vi "Process Image.vi"(8 "error in (no error)":errorcluster, 10 "Image Analysis IN":T1, 11 "Cluster in":T3={"Crosshair IN"={"Draw"=TRUE, "Target"={"x"=20.0, "y"=20.0}, "Size"={"x"=20.0, "y"=20.0}, "Angle"=1250067.0, "Color"=1250067, "Thickness"=20, "CrosshairLabel"=""}, "Autoscale"=FALSE, "Scale"={"scale factor"=0.0, "Scale"=FALSE}, "Lowpass IN"={"LowPass"=FALSE, "Size & Tolerance"={"X Size"=0, "Y Size"=0, "% Tolerance"=0}}, "Image"=refnum, "GUI_centroid overlay"={"CentroidX array"=[], "CentroidY array"=[], "CentroidX"=0.0, "CentroidY"=0.0, "# images to average"=1250067, "Crosshair"={"Draw"=TRUE, "Target"={"x"=20.0, "y"=20.0}, "Size"={"x"=20.0, "y"=20.0}, "Angle"=1250067.0, "Color"=1250067, "Thickness"=20, "CrosshairLabel"=""}}, "GUI Crosshair"={"Draw"=TRUE, "Target"={"x"=20.0, "y"=20.0}, "Size"={"x"=20.0, "y"=20.0}, "Angle"=1250067.0, "Color"=1250067, "Thickness"=20, "CrosshairLabel"=""}, "Crosshair2 IN"={"Draw"=TRUE, "Target"={"x"=20.0, "y"=20.0}, "Size"={"x"=20.0, "y"=20.0}, "Angle"=1250067.0, "Color"=1250067, "Thickness"=20, "CrosshairLabel"=""}} {"Crosshair2 IN"."Thickness" max=0; "Crosshair2 IN"."Target"."y" min=0.0 max=0.0; "Crosshair2 IN"."Target"."x" min=0.0 max=0.0; "Crosshair2 IN"."Angle" format="%#_13g"; "Crosshair2 IN"."Size"."y" min=0.0 max=0.0; "Crosshair2 IN"."Size"."x" min=0.0 max=0.0; "GUI Crosshair"."Thickness" max=0; "GUI Crosshair"."Target"."y" min=0.0 max=0.0; "GUI Crosshair"."Target"."x" min=0.0 max=0.0; "GUI Crosshair"."Angle" format="%#_13g"; "GUI Crosshair"."Size"."y" min=0.0 max=0.0; "GUI Crosshair"."Size"."x" min=0.0 max=0.0; "GUI_centroid overlay"."Crosshair"."Thickness" max=0; "GUI_centroid overlay"."Crosshair"."Target"."y" min=0.0 max=0.0; "GUI_centroid overlay"."Crosshair"."Target"."x" min=0.0 max=0.0; "GUI_centroid overlay"."Crosshair"."Angle" format="%#_13g"; "GUI_centroid overlay"."Crosshair"."Size"."y" min=0.0 max=0.0; "GUI_centroid overlay"."Crosshair"."Size"."x" min=0.0 max=0.0; "Crosshair IN"."Thickness" max=0; "Crosshair IN"."Target"."y" min=0.0 max=0.0; "Crosshair IN"."Target"."x" min=0.0 max=0.0; "Crosshair IN"."Angle" format="%#_13g"; "Crosshair IN"."Size"."y" min=0.0 max=0.0; "Crosshair IN"."Size"."x" min=0.0 max=0.0}) -> (0 "error out":errorcluster, 2 "Image Analysis OUT":T1, 3 "Cluster out":T3={"Crosshair IN"={"Draw"=TRUE, "Target"={"x"=20.0, "y"=20.0}, "Size"={"x"=20.0, "y"=20.0}, "Angle"=1250067.0, "Color"=1250067, "Thickness"=20, "CrosshairLabel"=""}, "Autoscale"=FALSE, "Scale"={"scale factor"=0.0, "Scale"=FALSE}, "Lowpass IN"={"LowPass"=FALSE, "Size & Tolerance"={"X Size"=0, "Y Size"=0, "% Tolerance"=0}}, "Image"=refnum, "GUI_centroid overlay"={"CentroidX array"=[], "CentroidY array"=[], "CentroidX"=0.0, "CentroidY"=0.0, "# images to average"=1250067, "Crosshair"={"Draw"=TRUE, "Target"={"x"=20.0, "y"=20.0}, "Size"={"x"=20.0, "y"=20.0}, "Angle"=1250067.0, "Color"=1250067, "Thickness"=20, "CrosshairLabel"=""}}, "GUI Crosshair"={"Draw"=TRUE, "Target"={"x"=20.0, "y"=20.0}, "Size"={"x"=20.0, "y"=20.0}, "Angle"=1250067.0, "Color"=1250067, "Thickness"=20, "CrosshairLabel"=""}, "Crosshair2 IN"={"Draw"=TRUE, "Target"={"x"=20.0, "y"=20.0}, "Size"={"x"=20.0, "y"=20.0}, "Angle"=1250067.0, "Color"=1250067, "Thickness"=20, "CrosshairLabel"=""}} {"Crosshair2 IN"."Thickness" max=0; "Crosshair2 IN"."Target"."y" min=0.0 max=0.0; "Crosshair2 IN"."Target"."x" min=0.0 max=0.0; "Crosshair2 IN"."Angle" format="%#_13g"; "Crosshair2 IN"."Size"."y" min=0.0 max=0.0; "Crosshair2 IN"."Size"."x" min=0.0 max=0.0; "GUI Crosshair"."Thickness" max=0; "GUI Crosshair"."Target"."y" min=0.0 max=0.0; "GUI Crosshair"."Target"."x" min=0.0 max=0.0; "GUI Crosshair"."Angle" format="%#_13g"; "GUI Crosshair"."Size"."y" min=0.0 max=0.0; "GUI Crosshair"."Size"."x" min=0.0 max=0.0; "GUI_centroid overlay"."Crosshair"."Thickness" max=0; "GUI_centroid overlay"."Crosshair"."Target"."y" min=0.0 max=0.0; "GUI_centroid overlay"."Crosshair"."Target"."x" min=0.0 max=0.0; "GUI_centroid overlay"."Crosshair"."Angle" format="%#_13g"; "GUI_centroid overlay"."Crosshair"."Size"."y" min=0.0 max=0.0; "GUI_centroid overlay"."Crosshair"."Size"."x" min=0.0 max=0.0; "Crosshair IN"."Thickness" max=0; "Crosshair IN"."Target"."y" min=0.0 max=0.0; "Crosshair IN"."Target"."x" min=0.0 max=0.0; "Crosshair IN"."Angle" format="%#_13g"; "Crosshair IN"."Size"."y" min=0.0 max=0.0; "Crosshair IN"."Size"."x" min=0.0 max=0.0})   [LabVIEW 2013]
uses:
  Controls/Image Processing Controls.ctl
  Controls/Crosshair type def.ctl
  <vilib>/vision/Image Controls.llb/IMAQ Image.ctl
  Controls/GUI_running average centroid overlay.ctl
  Controls/Image Analysis Controls.ctl
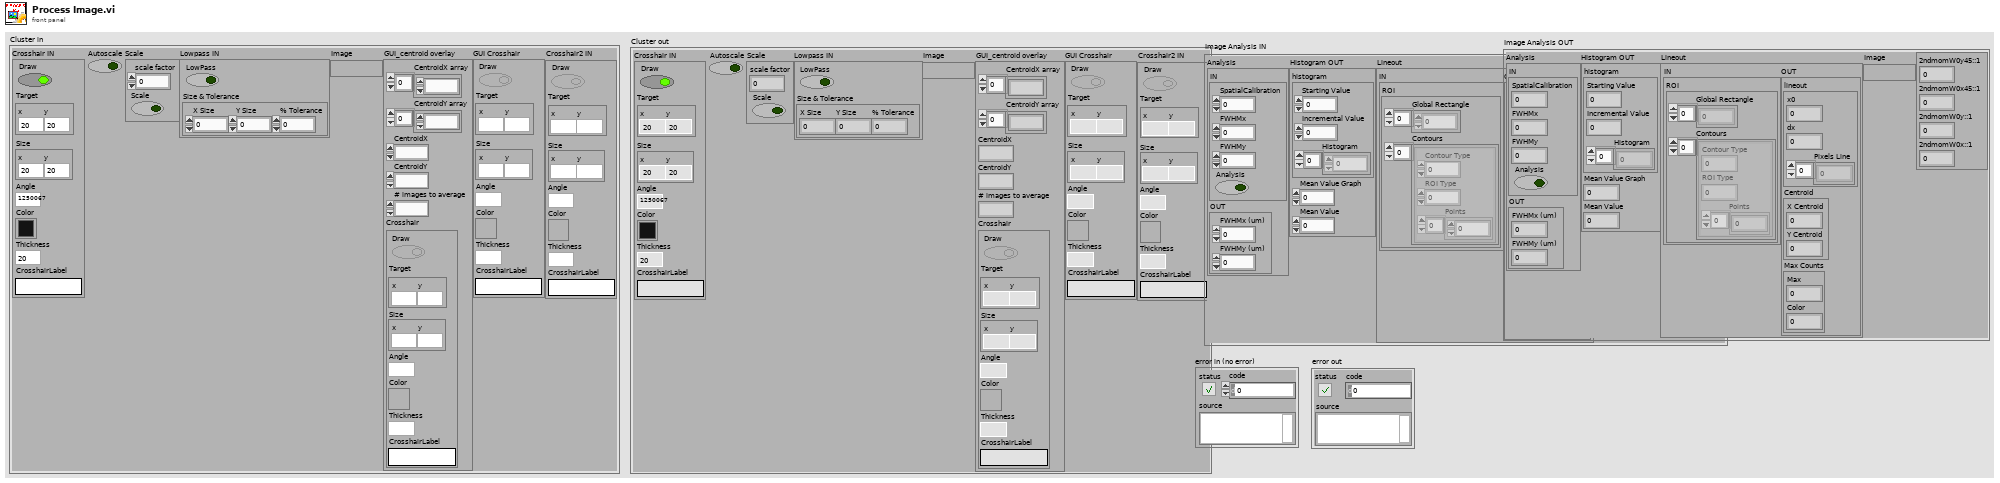
[diagram p1: front panel]
types:
  T1 = typedef "Image Analysis Controls.ctl" = cluster{"Analysis":cluster{"IN":cluster{"SpatialCalibration":dbl, "FWHMx":dbl, "FWHMy":dbl, "Analysis":bool}, "OUT":cluster{"FWHMx (um)":dbl, "FWHMy (um)":dbl}}, "Histogram OUT":cluster{"histogram":cluster{"Starting Value":sgl, "Incremental Value":sgl, "Histogram":u32[]}, "Mean Value Graph":sgl, "Mean Value":sgl}, "Lineout":cluster{"IN":cluster{"ROI":cluster{"Global Rectangle":i32[], "Contours":cluster{"Contour Type":u32, "ROI Type":u32, "Points":i32[]}[]}}, "OUT":cluster{"lineout":cluster{"x0":sgl, "dx":sgl, "Pixels Line":sgl[]}, "Centroid":cluster{"X Centroid":sgl, "Y Centroid":sgl}, "Max Counts":cluster{"Max":sgl, "Color":u32}}}, "Image":T2, "variables":cluster{"2ndmomW0y45::1":dbl, "2ndmomW0x45::1":dbl, "2ndmomW0y::1":dbl, "2ndmomW0x::1":dbl}}
  T2 = typedef "IMAQ Image.ctl" = refnum<image>
  T3 = typedef "Image Processing Controls.ctl" = cluster{"Crosshair IN":T4, "Autoscale":bool, "Scale":cluster{"scale factor":dbl, "Scale":bool}, "Lowpass IN":cluster{"LowPass":bool, "Size & Tolerance":cluster{"X Size":i32, "Y Size":i32, "% Tolerance":i32}}, "Image":T2, "GUI_centroid overlay":T5, "GUI Crosshair":T4, "Crosshair2 IN":T4}
  T4 = typedef "Crosshair type def.ctl" = cluster{"Draw":bool, "Target":cluster{"x":dbl, "y":dbl}, "Size":cluster{"x":dbl, "y":dbl}, "Angle":dbl, "Color":u32, "Thickness":u8, "CrosshairLabel":string}
  T5 = typedef "GUI_running average centroid overlay.ctl" = cluster{"CentroidX array":dbl[], "CentroidY array":dbl[], "CentroidX":dbl, "CentroidY":dbl, "# images to average":i32, "Crosshair":T4}
  T6 = cluster{"LowPass":bool, "Size & Tolerance":cluster{"X Size":i32, "Y Size":i32, "% Tolerance":i32}}
  T7 = cluster{"SpatialCalibration":dbl, "FWHMx":dbl, "FWHMy":dbl, "Analysis":bool}
  T8 = cluster{"ROI":cluster{"Global Rectangle":i32[], "Contours":cluster{"Contour Type":u32, "ROI Type":u32, "Points":i32[]}[]}}
  T9 = cluster{"histogram":cluster{"Starting Value":sgl, "Incremental Value":sgl, "Histogram":u32[]}, "Mean Value Graph":sgl, "Mean Value":sgl}
  T10 = cluster{"lineout":cluster{"x0":sgl, "dx":sgl, "Pixels Line":sgl[]}, "Centroid":cluster{"X Centroid":sgl, "Y Centroid":sgl}, "Max Counts":cluster{"Max Value":sgl, "Color":u32}}
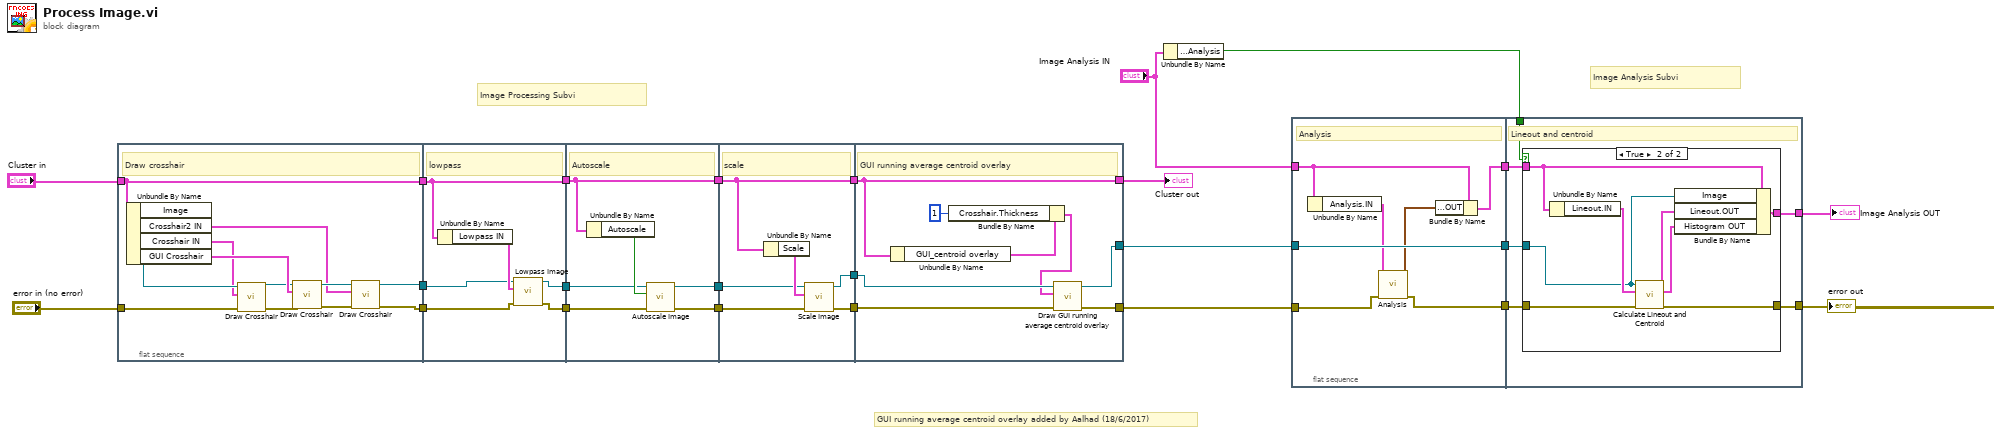
[diagram p0: block diagram]
diagram:
  # "GUI running average centroid overlay added by Aalhad (18/6/2017)"
  # "Image Analysis Subvi"
  # "Image Processing Subvi"
  n1 = flat-sequence {
    tunnel: [w36] -> w18
    tunnel: [w29] -> w17
    tunnel: [w27] -> w11
    tunnel: "Cluster in" -> [w36]
    tunnel: "error in (no error)" -> [w34]
    tunnel: [w41] -> w24
    tunnel: [w38] -> w23
    tunnel: w18 -> [w41]
    tunnel: w17 -> [w37]
    tunnel: w11 -> [w40]
    tunnel: [w39] -> w10
    tunnel: w24 -> [w43]
    tunnel: [w43] -> w22
    tunnel: w23 -> [w47]
    tunnel: [w46] -> w21
    tunnel: w10 -> [w44]
    tunnel: [w45] -> w9
    tunnel: w22 -> [w50]
    tunnel: w21 -> [w53]
    tunnel: w9 -> [w49]
    tunnel: [w50] -> w7
    tunnel: [w52] -> w6
    tunnel: [w51] -> w5
    tunnel: [w62] -> w15
    tunnel: [w61] -> w14
    tunnel: [w59] -> w20
    tunnel: w7 -> [w59]
    tunnel: w6 -> [w60]
    tunnel: w5 -> [w58]
    frame #0 {
      # "Draw crosshair"
      n2 = Unbundle By Name(w36) -> ("Image"=w35:T2, "Crosshair2 IN"=w25:T4, "Crosshair IN"=w26:T4, "GUI Crosshair"=w33:T4)
      n3 = call "Draw Crosshair.vi"("error in"=w34, "Crosshair"=w26, "Image in"=w35) -> ("error out"=w31:errorcluster, "image out"=w32:T2)  [unwired: 7 in]
      n4 = call "Draw Crosshair.vi"("error in"=w31, "Crosshair"=w33, "Image in"=w32) -> ("error out"=w30:errorcluster, "image out"=w28:T2)  [unwired: 7 in]
      n5 = call "Draw Crosshair.vi"("error in"=w30, "Crosshair"=w25, "Image in"=w28) -> ("error out"=w29:errorcluster, "image out"=w27:T2)  [unwired: 7 in]
    }
    frame #1 {
      # "lowpass"
      n6 = Unbundle By Name(w41) -> ("Lowpass IN"=w42:T6)
      n7 = call "Lowpass Image.vi"("error in"=w37, "Lowpass IN"=w42, "Refnum in"=w40) -> ("error out"=w38:errorcluster, "Refnum out"=w39:T2)  [unwired: 7 in]
    }
    frame #2 {
      # "Autoscale"
      n8 = Unbundle By Name(w43) -> ("Autoscale"=w48:bool)
      n9 = call "Autoscale Image.vi"("error in (no error)"=w47, "Autoscale"=w48, "Refnum in"=w44) -> ("error out"=w46:errorcluster, "Refnum out"=w45:T2)  [unwired: 7 in]
    }
    frame #3 {
      # "scale"
      n10 = Unbundle By Name(w50) -> ("Scale"=w54:cluster{"scale factor":dbl, "Scale":bool})
      n11 = call "Scale Image.vi"("error in (no error)"=w53, "Scale"=w54, "Refnum in"=w49) -> ("error out"=w52:errorcluster, "Refnum out"=w51:T2)  [unwired: 7 in]
    }
    frame #4 {
      # "GUI running average centroid overlay"
      n12 = Unbundle By Name(w59) -> ("GUI_centroid overlay"=w56:T5)
      n13 = Bundle By Name(cluster=w56, "Crosshair.Thickness"=u8 1) -> (w55:T5)
      n14 = call "Draw GUI running average centroid overlay.vi"("error in"=w60, "GUI_centroid overlay"=w55, "Image in"=w58) -> ("error out"=w61:errorcluster, "image out"=w62:T2)  [unwired: 7 in]
    }
  }
  n15 = Unbundle By Name("Image Analysis IN") -> ("Analysis.IN.Analysis"=w1:bool)
  n16 = flat-sequence {
    tunnel: w14 -> [w67]
    tunnel: w15 -> [w69]
    tunnel: "Image Analysis IN" -> [w65]
    tunnel: [w64] -> w4
    tunnel: [w69] -> w3
    tunnel: [w66] -> w2
    tunnel: w4 -> [w73]
    tunnel: w3 -> [w75]
    tunnel: w2 -> [w74]
    tunnel: [w72] -> w12
    tunnel: [w71] -> w13
    tunnel: w1 -> [w70]
    frame #0 {
      # "Analysis"
      n17 = Unbundle By Name(w65) -> ("Analysis.IN"=w68:T7)
      n18 = call "Analysis.vi"("error in"=w67, "IN"=w68) -> ("error out"=w66:errorcluster, "OUT"=w63:cluster{"FWHMx (um)":dbl, "FWHMy (um)":dbl})  [unwired: 8 in]
      n19 = Bundle By Name(cluster=w65, "Analysis.OUT"=w63) -> (w64:T1)
    }
    frame #1 {
      # "Lineout and centroid"
      n20 = case shown="True" w70 {
        tunnel: w75 -> [_ w83]
        tunnel: w74 -> [w77 w82]
        tunnel: w73 -> [w76 w81]
        tunnel: [w76 w79] -> w72
        tunnel: [w77 w78] -> w71
        frame False {
        }
        frame True {
          n21 = Unbundle By Name(w81) -> ("Lineout.IN"=w85:T8)
          n22 = call "Calculate Lineout and Centroid.vi"("error in (no error)"=w82, "Lineout IN"=w85, "Image"=w83) -> ("error out"=w78:errorcluster, "Histogram OUT"=w80:T9, "Lineout Out"=w84:T10)  [unwired: 6 in]
          n23 = Bundle By Name(cluster=w81, "Image"=w83, "Lineout.OUT"=w84, "Histogram OUT"=w80) -> (w79:T1)
        }
      }
    }
  }
  "Cluster out" <- w20
  "error out" <- w13
  "Image Analysis OUT" <- w12
